vi "request_scanner_delays.vi"(8 "error in (no error)":errorcluster, 11 "ScanHeadDL090202 in":refnum<class "ScanHeadDL090202.lvclass">) -> (0 "error out":errorcluster, 3 "ScanHeadDL090202 out":refnum<class "ScanHeadDL090202.lvclass">)   [LabVIEW 2010, in "ScanHeadDL090202.lvclass"]
uses:
  ScanHeadDL090202.lvclass
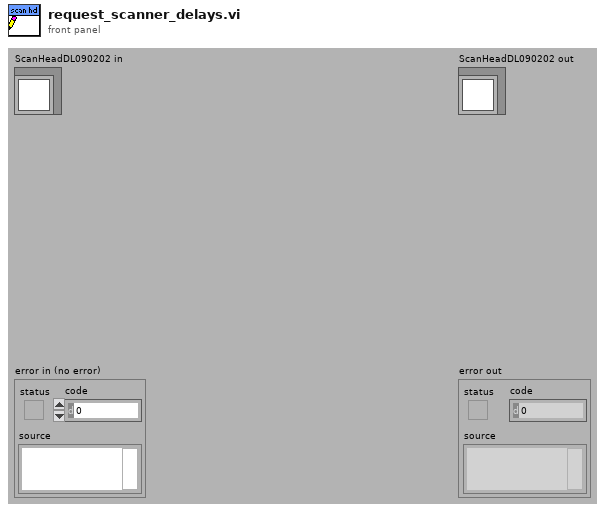
[diagram p1: front panel]
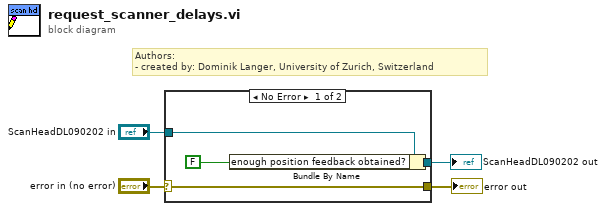
[diagram p0: block diagram]
diagram:
  # "Authors: \n- created by: Dominik Langer, University of Zurich, Switzerland"
  n1 = case shown="No Error" "error in (no error)" {
    selector: "error in (no error)" -> [w8 w9]
    tunnel: [w8 w9] -> w3
    tunnel: [w6 w10] -> w1
    tunnel: "ScanHeadDL090202 in" -> [w7 w10]
    frame No Error {
      n2 = Bundle By Name(cluster=w7, "enough position feedback obtained?"=FALSE) -> (w6:refnum<class "ScanHeadDL090202.lvclass">)
    }
    frame Error {
    }
  }
  "error out" <- w3
  "ScanHeadDL090202 out" <- w1
